vi "数字量输入配置.vi"() -> ()   [LabVIEW 2010] (continued)
                n7301 = property on="light_4" class="Bool (严格)"("Colors [4]"=w809) -> ()  [unwired: 2 in, 2 out]
                n7302 = property on="light_5" class="Bool (严格)"("Colors [4]"=w809) -> ()  [unwired: 2 in, 2 out]
                n7303 = property on="light_6" class="Bool (严格)"("Colors [4]"=w809) -> ()  [unwired: 2 in, 2 out]
                n7304 = property on="light_7" class="Bool (严格)"("Colors [4]"=w809) -> ()  [unwired: 2 in, 2 out]
                n7305 = property on="light_8" class="Bool (严格)"("Colors [4]"=w809) -> ()  [unwired: 2 in, 2 out]
                n7306 = property on="light_9" class="Bool (严格)"("Colors [4]"=w809) -> ()  [unwired: 2 in, 2 out]
                n7307 = property on="light_10" class="Bool (严格)"("Colors [4]"=w809) -> ()  [unwired: 2 in, 2 out]
                n7308 = property on="light_11" class="Bool (严格)"("Colors [4]"=w809) -> ()  [unwired: 2 in, 2 out]
                n7309 = property on="light_12" class="Bool (严格)"("Colors [4]"=w809) -> ()  [unwired: 2 in, 2 out]
                n7310 = property on="light_13" class="Bool (严格)"("Colors [4]"=w809) -> ()  [unwired: 2 in, 2 out]
                n7311 = property on="light_14" class="Bool (严格)"("Colors [4]"=w809) -> ()  [unwired: 2 in, 2 out]
                n7312 = property on="light_15" class="Bool (严格)"("Colors [4]"=w809) -> ()  [unwired: 2 in, 2 out]
                n7313 = property on="light_16" class="Bool (严格)"("Colors [4]"=w809) -> ()  [unwired: 2 in, 2 out]
                n7314 = property on="light_17" class="Bool (严格)"("Colors [4]"=w809) -> ()  [unwired: 2 in, 2 out]
                n7315 = property on="light_18" class="Bool (严格)"("Colors [4]"=w809) -> ()  [unwired: 2 in, 2 out]
                n7316 = property on="light_19" class="Bool (严格)"("Colors [4]"=w809) -> ()  [unwired: 2 in, 2 out]
                n7317 = property on="light_20" class="Bool (严格)"("Colors [4]"=w809) -> ()  [unwired: 2 in, 2 out]
                n7318 = property on="light_21" class="Bool (严格)"("Colors [4]"=w809) -> ()  [unwired: 2 in, 2 out]
                n7319 = property on="light_22" class="Bool (严格)"("Colors [4]"=w809) -> ()  [unwired: 2 in, 2 out]
                n7320 = property on="light_23" class="Bool (严格)"("Colors [4]"=w809) -> ()  [unwired: 2 in, 2 out]
                n7321 = property on="light_24" class="Bool (严格)"("Colors [4]"=w809) -> ()  [unwired: 2 in, 2 out]
                n7322 = property on="light_25" class="Bool (严格)"("Colors [4]"=w809) -> ()  [unwired: 2 in, 2 out]
                n7323 = property on="light_26" class="Bool (严格)"("Colors [4]"=w809) -> ()  [unwired: 2 in, 2 out]
                n7324 = property on="light_27" class="Bool (严格)"("Colors [4]"=w809) -> ()  [unwired: 2 in, 2 out]
                n7325 = property on="light_28" class="Bool (严格)"("Colors [4]"=w809) -> ()  [unwired: 2 in, 2 out]
                n7326 = property on="light_29" class="Bool (严格)"("Colors [4]"=w809) -> ()  [unwired: 2 in, 2 out]
                n7327 = property on="light_30" class="Bool (严格)"("Colors [4]"=w809) -> ()  [unwired: 2 in, 2 out]
                n7328 = property on="light_31" class="Bool (严格)"("Colors [4]"=w809) -> ()  [unwired: 2 in, 2 out]
                n7329 = property on="light_32" class="Bool (严格)"("Colors [4]"=w809) -> ()  [unwired: 2 in, 2 out]
                n7330 = property on="light_33" class="Bool (严格)"("Colors [4]"=w809) -> ()  [unwired: 2 in, 2 out]
                n7331 = property on="light_34" class="Bool (严格)"("Colors [4]"=w809) -> ()  [unwired: 2 in, 2 out]
                n7332 = property on="light_35" class="Bool (严格)"("Colors [4]"=w809) -> ()  [unwired: 2 in, 2 out]
                n7333 = property on="light_36" class="Bool (严格)"("Colors [4]"=w809) -> ()  [unwired: 2 in, 2 out]
                n7334 = property on="light_37" class="Bool (严格)"("Colors [4]"=w809) -> ()  [unwired: 2 in, 2 out]
                n7335 = property on="light_38" class="Bool (严格)"("Colors [4]"=w809) -> ()  [unwired: 2 in, 2 out]
                n7336 = property on="light_39" class="Bool (严格)"("Colors [4]"=w809) -> ()  [unwired: 2 in, 2 out]
                n7337 = property on="light_40" class="Bool (严格)"("Colors [4]"=w809) -> ()  [unwired: 2 in, 2 out]
                n7338 = property on="light_41" class="Bool (严格)"("Colors [4]"=w809) -> ()  [unwired: 2 in, 2 out]
                n7339 = property on="light_42" class="Bool (严格)"("Colors [4]"=w809) -> ()  [unwired: 2 in, 2 out]
                n7340 = property on="light_43" class="Bool (严格)"("Colors [4]"=w809) -> ()  [unwired: 2 in, 2 out]
                n7341 = property on="light_44" class="Bool (严格)"("Colors [4]"=w809) -> ()  [unwired: 2 in, 2 out]
                n7342 = property on="light_45" class="Bool (严格)"("Colors [4]"=w809) -> ()  [unwired: 2 in, 2 out]
                n7343 = property on="light_46" class="Bool (严格)"("Colors [4]"=w809) -> ()  [unwired: 2 in, 2 out]
                n7344 = property on="light_47" class="Bool (严格)"("Colors [4]"=w809) -> ()  [unwired: 2 in, 2 out]
                n7345 = property on="light_48" class="Bool (严格)"("Colors [4]"=w809) -> ()  [unwired: 2 in, 2 out]
                n7346 = property on="light_49" class="Bool (严格)"("Colors [4]"=w809) -> ()  [unwired: 2 in, 2 out]
                n7347 = property on="light_50" class="Bool (严格)"("Colors [4]"=w809) -> ()  [unwired: 2 in, 2 out]
                n7348 = property on="light_51" class="Bool (严格)"("Colors [4]"=w809) -> ()  [unwired: 2 in, 2 out]
                n7349 = property on="light_52" class="Bool (严格)"("Colors [4]"=w809) -> ()  [unwired: 2 in, 2 out]
                n7350 = property on="light_53" class="Bool (严格)"("Colors [4]"=w809) -> ()  [unwired: 2 in, 2 out]
                n7351 = property on="light_54" class="Bool (严格)"("Colors [4]"=w809) -> ()  [unwired: 2 in, 2 out]
                n7352 = property on="light_55" class="Bool (严格)"("Colors [4]"=w809) -> ()  [unwired: 2 in, 2 out]
                n7353 = property on="light_56" class="Bool (严格)"("Colors [4]"=w809) -> ()  [unwired: 2 in, 2 out]
                n7354 = property on="light_57" class="Bool (严格)"("Colors [4]"=w809) -> ()  [unwired: 2 in, 2 out]
                n7355 = property on="light_58" class="Bool (严格)"("Colors [4]"=w809) -> ()  [unwired: 2 in, 2 out]
                n7356 = property on="light_59" class="Bool (严格)"("Colors [4]"=w809) -> ()  [unwired: 2 in, 2 out]
                n7357 = property on="light_60" class="Bool (严格)"("Colors [4]"=w809) -> ()  [unwired: 2 in, 2 out]
                n7358 = property on="light_61" class="Bool (严格)"("Colors [4]"=w809) -> ()  [unwired: 2 in, 2 out]
                n7359 = property on="light_62" class="Bool (严格)"("Colors [4]"=w809) -> ()  [unwired: 2 in, 2 out]
                n7360 = property on="light_63" class="Bool (严格)"("Colors [4]"=w809) -> ()  [unwired: 2 in, 2 out]
                n7361 = property on="light_64" class="Bool (严格)"("Colors [4]"=w809) -> ()  [unwired: 2 in, 2 out]
                n7362 = property on="light_65" class="Bool (严格)"("Colors [4]"=w809) -> ()  [unwired: 2 in, 2 out]
                n7363 = property on="light_66" class="Bool (严格)"("Colors [4]"=w809) -> ()  [unwired: 2 in, 2 out]
                n7364 = property on="light_67" class="Bool (严格)"("Colors [4]"=w809) -> ()  [unwired: 2 in, 2 out]
                n7365 = property on="light_68" class="Bool (严格)"("Colors [4]"=w809) -> ()  [unwired: 2 in, 2 out]
                n7366 = property on="light_69" class="Bool (严格)"("Colors [4]"=w809) -> ()  [unwired: 2 in, 2 out]
                n7367 = property on="light_70" class="Bool (严格)"("Colors [4]"=w809) -> ()  [unwired: 2 in, 2 out]
                n7368 = property on="light_71" class="Bool (严格)"("Colors [4]"=w809) -> ()  [unwired: 2 in, 2 out]
                n7369 = property on="light_72" class="Bool (严格)"("Colors [4]"=w809) -> ()  [unwired: 2 in, 2 out]
                n7370 = property on="light_73" class="Bool (严格)"("Colors [4]"=w809) -> ()  [unwired: 2 in, 2 out]
                n7371 = property on="light_74" class="Bool (严格)"("Colors [4]"=w809) -> ()  [unwired: 2 in, 2 out]
                n7372 = property on="light_75" class="Bool (严格)"("Colors [4]"=w809) -> ()  [unwired: 2 in, 2 out]
                n7373 = property on="light_76" class="Bool (严格)"("Colors [4]"=w809) -> ()  [unwired: 2 in, 2 out]
                n7374 = property on="light_77" class="Bool (严格)"("Colors [4]"=w809) -> ()  [unwired: 2 in, 2 out]
                n7375 = property on="light_78" class="Bool (严格)"("Colors [4]"=w809) -> ()  [unwired: 2 in, 2 out]
                n7376 = property on="light_79" class="Bool (严格)"("Colors [4]"=w809) -> ()  [unwired: 2 in, 2 out]
                n7377 = property on="light_80" class="Bool (严格)"("Colors [4]"=w809) -> ()  [unwired: 2 in, 2 out]
                n7378 = Initialize Array("", 16 ("维数大小"), 4 ("维数大小")) -> (w808:string[][])
                n7379 = local write "D_IN_1"(w808) -> ()
                n7380 = local write "D_IN_2"(w808) -> ()
                n7381 = local write "D_IN_3"(w808) -> ()
                n7382 = local write "D_IN_4"(w808) -> ()
                n7383 = local write "D_IN_5"(w808) -> ()
              }
              frame #2 {
                n7384 = local read "保持输入"() -> (w810:bool)
                n7385 = case shown="假" w810 {
                  frame False {
                    n7386 = property on="保持输入" class="Bool (严格)"("DisabledEnum"=T1."Disabled and Grayed Out" ("禁用")) -> ()  [unwired: 2 in, 2 out]
                  }
                  frame True {
                    n7387 = local read "数组_选择?"() -> (w812:bool[][])
                    n7388 = for {
                      tunnel: w812 -> [w816] mode=indexing
                      i -> [w814]
                      stop <- w813 stop-if-true
                      n7389 = Or Array Elements(Boolean array=w816) -> (logical OR=w815:bool)
                      n7390 = case shown="真" w815 {
                        tunnel: w814 -> [_ w818]
                        tunnel: [FALSE w821] -> w813
                        frame False {
                        }
                        frame True {
                          n7391 = local write "同步_A1"(w818) -> ()
                          n7392 = Increment(x=w818) -> (x+1=w823:i32)
                          n7393 = Format Into String(format string="保持第%d组数据输入" ("格式字符串"), w823) -> (resulting string=w824:string)  [unwired: 2 in, 1 out]
                          n7394 = call "显示对话框信息2"("Message"=w824) -> ("是"=w819:bool)  [unwired: 9 in, 1 out]
                          n7395 = case shown="真" w819 {
                            tunnel: [FALSE w829] -> w821
                            tunnel: [T1."Enabled" ("禁用") w828] -> w820
                            tunnel: w818 -> [_ w827]
                            frame False {
                            }
                            frame True {
                              n7396 = stacked-sequence {
                                tunnel: [_ TRUE] -> w829
                                tunnel: [_ T1."Disabled and Grayed Out" ("禁用")] -> w828
                                tunnel: w827 -> [w830 _]
                                frame #0 {
                                n7397 = for {
                                N: 5 -> [_]
                                tunnel: w830 -> [w833]
                                i -> [w832]
                                n7398 = Not Equal?(x=w833, y=w832) -> (x != y?=w834:bool)
                                n7399 = case shown="真" w834 {
                                tunnel: w832 -> [_ w835]
                                frame False {
                                }
                                frame True {
                                n7400 = local read "数组_选择?"() -> (w839:bool[][])
                                n7401 = Initialize Array(FALSE, 16 ("维数大小")) -> (w836:bool[])
                                n7402 = Replace Array Subset(array=w839, new element=w836, index (row)=w835) -> (w840:bool[][])  [unwired: 1 in]
                                n7403 = local write "数组_选择?"(w840) -> ()
                                }
                                }
                                }
                                }
                                frame #1 {
                                }
                              }
                            }
                          }
                          n7404 = local write "保持输入"(w819) -> ()
                          n7405 = property on="btn_开始试验" class="Bool"("DisabledEnum"=w820) -> ()  [unwired: 2 in, 2 out]
                        }
                      }
                    }
                  }
                }
              }
              frame #3 {
                n7406 = local read "数组_选择?"() -> (w846:bool[][])
                n7407 = Or Array Elements(Boolean array=w846) -> (logical OR=w845:bool)
                n7408 = case shown="真" w845 {
                  tunnel: w844 -> [_ w849]
                  tunnel: w843 -> [_ w848]
                  frame False {
                    n7409 = call "显示对话框信息"("Message"="请选择数字量输入路数") -> ()  [unwired: 9 in, 2 out]
                  }
                  frame True {
                    n7410 = Send Notification(notification="DInput" ("通知"), notifier=w849, error in (no error)=w848) -> ()  [unwired: 2 out]
                  }
                }
              }
            }
          }
          event "保持输入": Value Change {
            n7411 = event-data() -> ()  [unwired: 1 in, 5 out]
            n7412 = property on="btn_开始试验" class="Bool"("DisabledEnum"=T1."Enabled" ("禁用")) -> ()  [unwired: 2 in, 2 out]
          }
          event "btn_全选": Value Change {
            w852 = TRUE ("单选_第41路")
            n7413 = event-data() -> ()  [unwired: 1 in, 5 out]
            n7414 = local write "单选_第1路"(w852) -> ()
            n7415 = local write "单选_第2路"(w852) -> ()
            n7416 = local write "单选_第3路"(w852) -> ()
            n7417 = local write "单选_第4路"(w852) -> ()
            n7418 = local write "单选_第5路"(w852) -> ()
            n7419 = local write "单选_第6路"(w852) -> ()
            n7420 = local write "单选_第7路"(w852) -> ()
            n7421 = local write "单选_第8路"(w852) -> ()
            n7422 = local write "单选_第9路"(w852) -> ()
            n7423 = local write "单选_第10路"(w852) -> ()
            n7424 = local write "单选_第11路"(w852) -> ()
            n7425 = local write "单选_第12路"(w852) -> ()
            n7426 = local write "单选_第13路"(w852) -> ()
            n7427 = local write "单选_第14路"(w852) -> ()
            n7428 = local write "单选_第15路"(w852) -> ()
            n7429 = local write "单选_第16路"(w852) -> ()
            n7430 = local write "单选_第17路"(w852) -> ()
            n7431 = local write "单选_第18路"(w852) -> ()
            n7432 = local write "单选_第19路"(w852) -> ()
            n7433 = local write "单选_第20路"(w852) -> ()
            n7434 = local write "单选_第21路"(w852) -> ()
            n7435 = local write "单选_第22路"(w852) -> ()
            n7436 = local write "单选_第23路"(w852) -> ()
            n7437 = local write "单选_第24路"(w852) -> ()
            n7438 = local write "单选_第25路"(w852) -> ()
            n7439 = local write "单选_第26路"(w852) -> ()
            n7440 = local write "单选_第27路"(w852) -> ()
            n7441 = local write "单选_第28路"(w852) -> ()
            n7442 = local write "单选_第29路"(w852) -> ()
            n7443 = local write "单选_第30路"(w852) -> ()
            n7444 = local write "单选_第31路"(w852) -> ()
            n7445 = local write "单选_第32路"(w852) -> ()
            n7446 = local write "单选_第33路"(w852) -> ()
            n7447 = local write "单选_第34路"(w852) -> ()
            n7448 = local write "单选_第35路"(w852) -> ()
            n7449 = local write "单选_第36路"(w852) -> ()
            n7450 = local write "单选_第37路"(w852) -> ()
            n7451 = local write "单选_第38路"(w852) -> ()
            n7452 = local write "单选_第39路"(w852) -> ()
            n7453 = local write "单选_第40路"(w852) -> ()
            n7454 = local write "单选_第41路"(w852) -> ()
            n7455 = local write "单选_第42路"(w852) -> ()
            n7456 = local write "单选_第43路"(w852) -> ()
            n7457 = local write "单选_第44路"(w852) -> ()
            n7458 = local write "单选_第45路"(w852) -> ()
            n7459 = local write "单选_第46路"(w852) -> ()
            n7460 = local write "单选_第47路"(w852) -> ()
            n7461 = local write "单选_第48路"(w852) -> ()
            n7462 = local write "单选_第49路"(w852) -> ()
            n7463 = local write "单选_第50路"(w852) -> ()
            n7464 = local write "单选_第51路"(w852) -> ()
            n7465 = local write "单选_第52路"(w852) -> ()
            n7466 = local write "单选_第53路"(w852) -> ()
            n7467 = local write "单选_第54路"(w852) -> ()
            n7468 = local write "单选_第55路"(w852) -> ()
            n7469 = local write "单选_第56路"(w852) -> ()
            n7470 = local write "单选_第57路"(w852) -> ()
            n7471 = local write "单选_第58路"(w852) -> ()
            n7472 = local write "单选_第59路"(w852) -> ()
            n7473 = local write "单选_第60路"(w852) -> ()
            n7474 = local write "单选_第61路"(w852) -> ()
            n7475 = local write "单选_第62路"(w852) -> ()
            n7476 = local write "单选_第63路"(w852) -> ()
            n7477 = local write "单选_第64路"(w852) -> ()
            n7478 = local write "单选_第71路"(w852) -> ()
            n7479 = local write "单选_第79路"(w852) -> ()
            n7480 = local write "单选_第65路"(w852) -> ()
            n7481 = local write "单选_第66路"(w852) -> ()
            n7482 = local write "单选_第67路"(w852) -> ()
            n7483 = local write "单选_第68路"(w852) -> ()
            n7484 = local write "单选_第69路"(w852) -> ()
            n7485 = local write "单选_第70路"(w852) -> ()
            n7486 = local write "单选_第72路"(w852) -> ()
            n7487 = local write "单选_第73路"(w852) -> ()
            n7488 = local write "单选_第74路"(w852) -> ()
            n7489 = local write "单选_第75路"(w852) -> ()
            n7490 = local write "单选_第76路"(w852) -> ()
            n7491 = local write "单选_第77路"(w852) -> ()
            n7492 = local write "单选_第78路"(w852) -> ()
            n7493 = local write "单选_第80路"(w852) -> ()
          }
          event "btn_反选": Value Change {
            n7494 = event-data() -> ()  [unwired: 1 in, 5 out]
            n7495 = local read "单选_第1路"() -> (w1012:bool)
            n7496 = local read "单选_第2路"() -> (w1010:bool)
            n7497 = local read "单选_第3路"() -> (w1008:bool)
            n7498 = local read "单选_第4路"() -> (w1006:bool)
            n7499 = local read "单选_第5路"() -> (w1004:bool)
            n7500 = local read "单选_第6路"() -> (w1002:bool)
            n7501 = local read "单选_第7路"() -> (w1001:bool)
            n7502 = local read "单选_第8路"() -> (w1000:bool)
            n7503 = local read "单选_第9路"() -> (w999:bool)
            n7504 = local read "单选_第10路"() -> (w998:bool)
            n7505 = local read "单选_第11路"() -> (w997:bool)
            n7506 = local read "单选_第12路"() -> (w996:bool)
            n7507 = local read "单选_第13路"() -> (w995:bool)
            n7508 = local read "单选_第14路"() -> (w994:bool)
            n7509 = local read "单选_第15路"() -> (w993:bool)
            n7510 = local read "单选_第16路"() -> (w992:bool)
            n7511 = local read "单选_第17路"() -> (w991:bool)
            n7512 = local read "单选_第18路"() -> (w990:bool)
            n7513 = local read "单选_第19路"() -> (w989:bool)
            n7514 = local read "单选_第20路"() -> (w988:bool)
            n7515 = local read "单选_第21路"() -> (w987:bool)
            n7516 = local read "单选_第22路"() -> (w986:bool)
            n7517 = local read "单选_第23路"() -> (w985:bool)
            n7518 = local read "单选_第24路"() -> (w984:bool)
            n7519 = local read "单选_第25路"() -> (w983:bool)
            n7520 = local read "单选_第26路"() -> (w982:bool)
            n7521 = local read "单选_第27路"() -> (w981:bool)
            n7522 = local read "单选_第28路"() -> (w980:bool)
            n7523 = local read "单选_第29路"() -> (w979:bool)
            n7524 = local read "单选_第30路"() -> (w978:bool)
            n7525 = local read "单选_第31路"() -> (w977:bool)
            n7526 = local read "单选_第32路"() -> (w976:bool)
            n7527 = local read "单选_第33路"() -> (w975:bool)
            n7528 = local read "单选_第34路"() -> (w974:bool)
            n7529 = local read "单选_第35路"() -> (w973:bool)
            n7530 = local read "单选_第36路"() -> (w972:bool)
            n7531 = local read "单选_第37路"() -> (w971:bool)
            n7532 = local read "单选_第38路"() -> (w970:bool)
            n7533 = local read "单选_第39路"() -> (w969:bool)
            n7534 = local read "单选_第40路"() -> (w968:bool)
            n7535 = Not(x=w1012) -> (.not. x?=w1011:bool)
            n7536 = Not(x=w1010) -> (.not. x?=w1009:bool)
            n7537 = Not(x=w1008) -> (.not. x?=w1007:bool)
            n7538 = Not(x=w1006) -> (.not. x?=w1005:bool)
            n7539 = Not(x=w1004) -> (.not. x?=w1003:bool)
            n7540 = Not(x=w1002) -> (.not. x?=w967:bool)
            n7541 = Not(x=w1001) -> (.not. x?=w966:bool)
            n7542 = Not(x=w1000) -> (.not. x?=w965:bool)
            n7543 = Not(x=w999) -> (.not. x?=w964:bool)
            n7544 = Not(x=w998) -> (.not. x?=w963:bool)
            n7545 = Not(x=w997) -> (.not. x?=w962:bool)
            n7546 = Not(x=w996) -> (.not. x?=w961:bool)
            n7547 = Not(x=w995) -> (.not. x?=w960:bool)
            n7548 = Not(x=w994) -> (.not. x?=w959:bool)
            n7549 = Not(x=w993) -> (.not. x?=w958:bool)
            n7550 = Not(x=w992) -> (.not. x?=w957:bool)
            n7551 = Not(x=w991) -> (.not. x?=w956:bool)
            n7552 = Not(x=w990) -> (.not. x?=w955:bool)
            n7553 = Not(x=w989) -> (.not. x?=w954:bool)
            n7554 = Not(x=w988) -> (.not. x?=w953:bool)
            n7555 = Not(x=w987) -> (.not. x?=w952:bool)
            n7556 = Not(x=w986) -> (.not. x?=w951:bool)
            n7557 = Not(x=w985) -> (.not. x?=w950:bool)
            n7558 = Not(x=w984) -> (.not. x?=w949:bool)
            n7559 = Not(x=w983) -> (.not. x?=w948:bool)
            n7560 = Not(x=w982) -> (.not. x?=w947:bool)
            n7561 = Not(x=w981) -> (.not. x?=w946:bool)
            n7562 = Not(x=w980) -> (.not. x?=w945:bool)
            n7563 = Not(x=w979) -> (.not. x?=w944:bool)
            n7564 = Not(x=w978) -> (.not. x?=w943:bool)
            n7565 = Not(x=w977) -> (.not. x?=w942:bool)
            n7566 = Not(x=w976) -> (.not. x?=w941:bool)
            n7567 = Not(x=w975) -> (.not. x?=w940:bool)
            n7568 = Not(x=w974) -> (.not. x?=w939:bool)
            n7569 = Not(x=w973) -> (.not. x?=w938:bool)
            n7570 = Not(x=w972) -> (.not. x?=w937:bool)
            n7571 = Not(x=w971) -> (.not. x?=w936:bool)
            n7572 = Not(x=w970) -> (.not. x?=w935:bool)
            n7573 = Not(x=w969) -> (.not. x?=w934:bool)
            n7574 = Not(x=w968) -> (.not. x?=w933:bool)
            n7575 = local write "单选_第1路"(w1011) -> ()
            n7576 = local write "单选_第2路"(w1009) -> ()
            n7577 = local write "单选_第3路"(w1007) -> ()
            n7578 = local write "单选_第4路"(w1005) -> ()
            n7579 = local write "单选_第5路"(w1003) -> ()
            n7580 = local write "单选_第6路"(w967) -> ()
            n7581 = local write "单选_第7路"(w966) -> ()
            n7582 = local write "单选_第8路"(w965) -> ()
            n7583 = local write "单选_第9路"(w964) -> ()
            n7584 = local write "单选_第10路"(w963) -> ()
            n7585 = local write "单选_第11路"(w962) -> ()
            n7586 = local write "单选_第12路"(w961) -> ()
            n7587 = local write "单选_第13路"(w960) -> ()
            n7588 = local write "单选_第14路"(w959) -> ()
            n7589 = local write "单选_第15路"(w958) -> ()
            n7590 = local write "单选_第16路"(w957) -> ()
            n7591 = local write "单选_第17路"(w956) -> ()
            n7592 = local write "单选_第18路"(w955) -> ()
            n7593 = local write "单选_第19路"(w954) -> ()
            n7594 = local write "单选_第20路"(w953) -> ()
            n7595 = local write "单选_第21路"(w952) -> ()
            n7596 = local write "单选_第22路"(w951) -> ()
            n7597 = local write "单选_第23路"(w950) -> ()
            n7598 = local write "单选_第24路"(w949) -> ()
            n7599 = local write "单选_第25路"(w948) -> ()
            n7600 = local write "单选_第26路"(w947) -> ()
            n7601 = local write "单选_第27路"(w946) -> ()
            n7602 = local write "单选_第28路"(w945) -> ()
            n7603 = local write "单选_第29路"(w944) -> ()
            n7604 = local write "单选_第30路"(w943) -> ()
            n7605 = local write "单选_第31路"(w942) -> ()
            n7606 = local write "单选_第32路"(w941) -> ()
            n7607 = local write "单选_第33路"(w940) -> ()
            n7608 = local write "单选_第34路"(w939) -> ()
            n7609 = local write "单选_第35路"(w938) -> ()
            n7610 = local write "单选_第36路"(w937) -> ()
            n7611 = local write "单选_第37路"(w936) -> ()
            n7612 = local write "单选_第38路"(w935) -> ()
            n7613 = local write "单选_第39路"(w934) -> ()
            n7614 = local write "单选_第40路"(w933) -> ()
            n7615 = local read "单选_第71路"() -> (w902:bool)
            n7616 = local read "单选_第79路"() -> (w894:bool)
            n7617 = local read "单选_第41路"() -> (w932:bool)
            n7618 = local read "单选_第42路"() -> (w931:bool)
            n7619 = local read "单选_第43路"() -> (w930:bool)
            n7620 = local read "单选_第44路"() -> (w929:bool)
            n7621 = local read "单选_第45路"() -> (w928:bool)
            n7622 = local read "单选_第46路"() -> (w927:bool)
            n7623 = local read "单选_第47路"() -> (w926:bool)
            n7624 = local read "单选_第48路"() -> (w925:bool)
            n7625 = local read "单选_第49路"() -> (w924:bool)
            n7626 = local read "单选_第50路"() -> (w923:bool)
            n7627 = local read "单选_第51路"() -> (w922:bool)
            n7628 = local read "单选_第52路"() -> (w921:bool)
            n7629 = local read "单选_第53路"() -> (w920:bool)
            n7630 = local read "单选_第54路"() -> (w919:bool)
            n7631 = local read "单选_第55路"() -> (w918:bool)
            n7632 = local read "单选_第56路"() -> (w917:bool)
            n7633 = local read "单选_第57路"() -> (w916:bool)
            n7634 = local read "单选_第58路"() -> (w915:bool)
            n7635 = local read "单选_第59路"() -> (w914:bool)
            n7636 = local read "单选_第60路"() -> (w913:bool)
            n7637 = local read "单选_第61路"() -> (w912:bool)
            n7638 = local read "单选_第62路"() -> (w911:bool)
            n7639 = local read "单选_第63路"() -> (w910:bool)
            n7640 = local read "单选_第64路"() -> (w909:bool)
            n7641 = local read "单选_第65路"() -> (w908:bool)
            n7642 = local read "单选_第66路"() -> (w907:bool)
            n7643 = local read "单选_第67路"() -> (w906:bool)
            n7644 = local read "单选_第68路"() -> (w905:bool)
            n7645 = local read "单选_第69路"() -> (w904:bool)
            n7646 = local read "单选_第70路"() -> (w903:bool)
            n7647 = local read "单选_第72路"() -> (w901:bool)
            n7648 = local read "单选_第73路"() -> (w900:bool)
            n7649 = local read "单选_第74路"() -> (w899:bool)
            n7650 = local read "单选_第75路"() -> (w898:bool)
            n7651 = local read "单选_第76路"() -> (w897:bool)
            n7652 = local read "单选_第77路"() -> (w896:bool)
            n7653 = local read "单选_第78路"() -> (w895:bool)
            n7654 = local read "单选_第80路"() -> (w893:bool)
            n7655 = Not(x=w932) -> (.not. x?=w892:bool)
            n7656 = Not(x=w931) -> (.not. x?=w891:bool)
            n7657 = Not(x=w930) -> (.not. x?=w890:bool)
            n7658 = Not(x=w929) -> (.not. x?=w889:bool)
            n7659 = Not(x=w928) -> (.not. x?=w888:bool)
            n7660 = Not(x=w927) -> (.not. x?=w887:bool)
            n7661 = Not(x=w926) -> (.not. x?=w886:bool)
            n7662 = Not(x=w925) -> (.not. x?=w885:bool)
            n7663 = Not(x=w924) -> (.not. x?=w884:bool)
            n7664 = Not(x=w923) -> (.not. x?=w883:bool)
            n7665 = Not(x=w922) -> (.not. x?=w882:bool)
            n7666 = Not(x=w921) -> (.not. x?=w881:bool)
            n7667 = Not(x=w920) -> (.not. x?=w880:bool)
            n7668 = Not(x=w919) -> (.not. x?=w879:bool)
            n7669 = Not(x=w918) -> (.not. x?=w878:bool)
            n7670 = Not(x=w917) -> (.not. x?=w877:bool)
            n7671 = Not(x=w916) -> (.not. x?=w876:bool)
            n7672 = Not(x=w915) -> (.not. x?=w875:bool)
            n7673 = Not(x=w914) -> (.not. x?=w874:bool)
            n7674 = Not(x=w913) -> (.not. x?=w873:bool)
            n7675 = Not(x=w912) -> (.not. x?=w872:bool)
            n7676 = Not(x=w911) -> (.not. x?=w871:bool)
            n7677 = Not(x=w910) -> (.not. x?=w870:bool)
            n7678 = Not(x=w909) -> (.not. x?=w869:bool)
            n7679 = Not(x=w908) -> (.not. x?=w868:bool)
            n7680 = Not(x=w907) -> (.not. x?=w867:bool)
            n7681 = Not(x=w906) -> (.not. x?=w866:bool)
            n7682 = Not(x=w905) -> (.not. x?=w865:bool)
            n7683 = Not(x=w904) -> (.not. x?=w864:bool)
            n7684 = Not(x=w903) -> (.not. x?=w863:bool)
            n7685 = Not(x=w902) -> (.not. x?=w862:bool)
            n7686 = Not(x=w901) -> (.not. x?=w861:bool)
            n7687 = Not(x=w900) -> (.not. x?=w860:bool)
            n7688 = Not(x=w899) -> (.not. x?=w859:bool)
            n7689 = Not(x=w898) -> (.not. x?=w858:bool)
            n7690 = Not(x=w897) -> (.not. x?=w857:bool)
            n7691 = Not(x=w896) -> (.not. x?=w856:bool)
            n7692 = Not(x=w895) -> (.not. x?=w855:bool)
            n7693 = Not(x=w894) -> (.not. x?=w854:bool)
            n7694 = Not(x=w893) -> (.not. x?=w853:bool)
            n7695 = local write "单选_第71路"(w862) -> ()
            n7696 = local write "单选_第79路"(w854) -> ()
            n7697 = local write "单选_第41路"(w892) -> ()
            n7698 = local write "单选_第42路"(w891) -> ()
            n7699 = local write "单选_第43路"(w890) -> ()
            n7700 = local write "单选_第44路"(w889) -> ()
            n7701 = local write "单选_第45路"(w888) -> ()
            n7702 = local write "单选_第46路"(w887) -> ()
            n7703 = local write "单选_第47路"(w886) -> ()
            n7704 = local write "单选_第48路"(w885) -> ()
            n7705 = local write "单选_第49路"(w884) -> ()
            n7706 = local write "单选_第50路"(w883) -> ()
            n7707 = local write "单选_第51路"(w882) -> ()
            n7708 = local write "单选_第52路"(w881) -> ()
            n7709 = local write "单选_第53路"(w880) -> ()
            n7710 = local write "单选_第54路"(w879) -> ()
            n7711 = local write "单选_第55路"(w878) -> ()
            n7712 = local write "单选_第56路"(w877) -> ()
            n7713 = local write "单选_第57路"(w876) -> ()
            n7714 = local write "单选_第58路"(w875) -> ()
            n7715 = local write "单选_第59路"(w874) -> ()
            n7716 = local write "单选_第60路"(w873) -> ()
            n7717 = local write "单选_第61路"(w872) -> ()
            n7718 = local write "单选_第62路"(w871) -> ()
            n7719 = local write "单选_第63路"(w870) -> ()
            n7720 = local write "单选_第64路"(w869) -> ()
            n7721 = local write "单选_第65路"(w868) -> ()
            n7722 = local write "单选_第66路"(w867) -> ()
            n7723 = local write "单选_第67路"(w866) -> ()
            n7724 = local write "单选_第68路"(w865) -> ()
            n7725 = local write "单选_第69路"(w864) -> ()
            n7726 = local write "单选_第70路"(w863) -> ()
            n7727 = local write "单选_第72路"(w861) -> ()
            n7728 = local write "单选_第73路"(w860) -> ()
            n7729 = local write "单选_第74路"(w859) -> ()
            n7730 = local write "单选_第75路"(w858) -> ()
            n7731 = local write "单选_第76路"(w857) -> ()
            n7732 = local write "单选_第77路"(w856) -> ()
            n7733 = local write "单选_第78路"(w855) -> ()
            n7734 = local write "单选_第80路"(w853) -> ()
          }
          event "btn_置1": Value Change {
            w1013 = enum16{"0", "1"}."1" ("输入值_41")
            n7735 = event-data() -> ()  [unwired: 1 in, 5 out]
            n7736 = local write "输入值_1"(w1013) -> ()
            n7737 = local write "输入值_2"(w1013) -> ()
            n7738 = local write "输入值_3"(w1013) -> ()
            n7739 = local write "输入值_4"(w1013) -> ()
            n7740 = local write "输入值_5"(w1013) -> ()
            n7741 = local write "输入值_6"(w1013) -> ()
            n7742 = local write "输入值_7"(w1013) -> ()
            n7743 = local write "输入值_8"(w1013) -> ()
            n7744 = local write "输入值_9"(w1013) -> ()
            n7745 = local write "输入值_10"(w1013) -> ()
            n7746 = local write "输入值_11"(w1013) -> ()
            n7747 = local write "输入值_12"(w1013) -> ()
            n7748 = local write "输入值_13"(w1013) -> ()
            n7749 = local write "输入值_14"(w1013) -> ()
            n7750 = local write "输入值_15"(w1013) -> ()
            n7751 = local write "输入值_16"(w1013) -> ()
            n7752 = local write "输入值_17"(w1013) -> ()
            n7753 = local write "输入值_18"(w1013) -> ()
            n7754 = local write "输入值_19"(w1013) -> ()
            n7755 = local write "输入值_20"(w1013) -> ()
            n7756 = local write "输入值_21"(w1013) -> ()
            n7757 = local write "输入值_22"(w1013) -> ()
            n7758 = local write "输入值_23"(w1013) -> ()
            n7759 = local write "输入值_24"(w1013) -> ()
            n7760 = local write "输入值_25"(w1013) -> ()
            n7761 = local write "输入值_26"(w1013) -> ()
            n7762 = local write "输入值_27"(w1013) -> ()
            n7763 = local write "输入值_28"(w1013) -> ()
            n7764 = local write "输入值_29"(w1013) -> ()
            n7765 = local write "输入值_30"(w1013) -> ()
            n7766 = local write "输入值_31"(w1013) -> ()
            n7767 = local write "输入值_32"(w1013) -> ()
            n7768 = local write "输入值_33"(w1013) -> ()
            n7769 = local write "输入值_34"(w1013) -> ()
            n7770 = local write "输入值_35"(w1013) -> ()
            n7771 = local write "输入值_36"(w1013) -> ()
            n7772 = local write "输入值_37"(w1013) -> ()
            n7773 = local write "输入值_38"(w1013) -> ()
            n7774 = local write "输入值_39"(w1013) -> ()
            n7775 = local write "输入值_40"(w1013) -> ()
            n7776 = local write "输入值_41"(w1013) -> ()
            n7777 = local write "输入值_42"(w1013) -> ()
            n7778 = local write "输入值_43"(w1013) -> ()
            n7779 = local write "输入值_44"(w1013) -> ()
            n7780 = local write "输入值_45"(w1013) -> ()
            n7781 = local write "输入值_46"(w1013) -> ()
            n7782 = local write "输入值_47"(w1013) -> ()
            n7783 = local write "输入值_48"(w1013) -> ()
            n7784 = local write "输入值_49"(w1013) -> ()
            n7785 = local write "输入值_50"(w1013) -> ()
            n7786 = local write "输入值_51"(w1013) -> ()
            n7787 = local write "输入值_52"(w1013) -> ()
            n7788 = local write "输入值_53"(w1013) -> ()
            n7789 = local write "输入值_54"(w1013) -> ()
            n7790 = local write "输入值_55"(w1013) -> ()
            n7791 = local write "输入值_56"(w1013) -> ()
            n7792 = local write "输入值_57"(w1013) -> ()
            n7793 = local write "输入值_58"(w1013) -> ()
            n7794 = local write "输入值_59"(w1013) -> ()
            n7795 = local write "输入值_60"(w1013) -> ()
            n7796 = local write "输入值_61"(w1013) -> ()
            n7797 = local write "输入值_62"(w1013) -> ()
            n7798 = local write "输入值_63"(w1013) -> ()
            n7799 = local write "输入值_64"(w1013) -> ()
            n7800 = local write "输入值_65"(w1013) -> ()
            n7801 = local write "输入值_66"(w1013) -> ()
            n7802 = local write "输入值_67"(w1013) -> ()
            n7803 = local write "输入值_68"(w1013) -> ()
            n7804 = local write "输入值_69"(w1013) -> ()
            n7805 = local write "输入值_70"(w1013) -> ()
            n7806 = local write "输入值_71"(w1013) -> ()
            n7807 = local write "输入值_72"(w1013) -> ()
            n7808 = local write "输入值_73"(w1013) -> ()
            n7809 = local write "输入值_74"(w1013) -> ()
            n7810 = local write "输入值_75"(w1013) -> ()
            n7811 = local write "输入值_76"(w1013) -> ()
            n7812 = local write "输入值_77"(w1013) -> ()
            n7813 = local write "输入值_78"(w1013) -> ()
            n7814 = local write "输入值_79"(w1013) -> ()
            n7815 = local write "输入值_80"(w1013) -> ()
          }
          event "btn_置0": Value Change {
            w1014 = enum16{"0", "1"}."0" ("输入值_41")
            n7816 = event-data() -> ()  [unwired: 1 in, 5 out]
            n7817 = local write "输入值_1"(w1014) -> ()
            n7818 = local write "输入值_2"(w1014) -> ()
            n7819 = local write "输入值_3"(w1014) -> ()
            n7820 = local write "输入值_4"(w1014) -> ()
            n7821 = local write "输入值_5"(w1014) -> ()
            n7822 = local write "输入值_6"(w1014) -> ()
            n7823 = local write "输入值_7"(w1014) -> ()
            n7824 = local write "输入值_8"(w1014) -> ()
            n7825 = local write "输入值_9"(w1014) -> ()
            n7826 = local write "输入值_10"(w1014) -> ()
            n7827 = local write "输入值_11"(w1014) -> ()
            n7828 = local write "输入值_12"(w1014) -> ()
            n7829 = local write "输入值_13"(w1014) -> ()
            n7830 = local write "输入值_14"(w1014) -> ()
            n7831 = local write "输入值_15"(w1014) -> ()
            n7832 = local write "输入值_16"(w1014) -> ()
            n7833 = local write "输入值_17"(w1014) -> ()
            n7834 = local write "输入值_18"(w1014) -> ()
            n7835 = local write "输入值_19"(w1014) -> ()
            n7836 = local write "输入值_20"(w1014) -> ()
            n7837 = local write "输入值_21"(w1014) -> ()
            n7838 = local write "输入值_22"(w1014) -> ()
            n7839 = local write "输入值_23"(w1014) -> ()
            n7840 = local write "输入值_24"(w1014) -> ()
            n7841 = local write "输入值_25"(w1014) -> ()
            n7842 = local write "输入值_26"(w1014) -> ()
            n7843 = local write "输入值_27"(w1014) -> ()
            n7844 = local write "输入值_28"(w1014) -> ()
            n7845 = local write "输入值_29"(w1014) -> ()
            n7846 = local write "输入值_30"(w1014) -> ()
            n7847 = local write "输入值_31"(w1014) -> ()
            n7848 = local write "输入值_32"(w1014) -> ()
            n7849 = local write "输入值_33"(w1014) -> ()
            n7850 = local write "输入值_34"(w1014) -> ()
            n7851 = local write "输入值_35"(w1014) -> ()
            n7852 = local write "输入值_36"(w1014) -> ()
            n7853 = local write "输入值_37"(w1014) -> ()
            n7854 = local write "输入值_38"(w1014) -> ()
            n7855 = local write "输入值_39"(w1014) -> ()
            n7856 = local write "输入值_40"(w1014) -> ()
            n7857 = local write "输入值_41"(w1014) -> ()
            n7858 = local write "输入值_42"(w1014) -> ()
            n7859 = local write "输入值_43"(w1014) -> ()
            n7860 = local write "输入值_44"(w1014) -> ()
            n7861 = local write "输入值_45"(w1014) -> ()
            n7862 = local write "输入值_46"(w1014) -> ()
            n7863 = local write "输入值_47"(w1014) -> ()
            n7864 = local write "输入值_48"(w1014) -> ()
            n7865 = local write "输入值_49"(w1014) -> ()
            n7866 = local write "输入值_50"(w1014) -> ()
            n7867 = local write "输入值_51"(w1014) -> ()
            n7868 = local write "输入值_52"(w1014) -> ()
            n7869 = local write "输入值_53"(w1014) -> ()
            n7870 = local write "输入值_54"(w1014) -> ()
            n7871 = local write "输入值_55"(w1014) -> ()
            n7872 = local write "输入值_56"(w1014) -> ()
            n7873 = local write "输入值_57"(w1014) -> ()
            n7874 = local write "输入值_58"(w1014) -> ()
            n7875 = local write "输入值_59"(w1014) -> ()
            n7876 = local write "输入值_60"(w1014) -> ()
            n7877 = local write "输入值_61"(w1014) -> ()
            n7878 = local write "输入值_62"(w1014) -> ()
            n7879 = local write "输入值_63"(w1014) -> ()
            n7880 = local write "输入值_64"(w1014) -> ()
            n7881 = local write "输入值_65"(w1014) -> ()
            n7882 = local write "输入值_66"(w1014) -> ()
            n7883 = local write "输入值_67"(w1014) -> ()
            n7884 = local write "输入值_68"(w1014) -> ()
            n7885 = local write "输入值_69"(w1014) -> ()
            n7886 = local write "输入值_70"(w1014) -> ()
            n7887 = local write "输入值_71"(w1014) -> ()
            n7888 = local write "输入值_72"(w1014) -> ()
            n7889 = local write "输入值_73"(w1014) -> ()
            n7890 = local write "输入值_74"(w1014) -> ()
            n7891 = local write "输入值_75"(w1014) -> ()
            n7892 = local write "输入值_76"(w1014) -> ()
            n7893 = local write "输入值_77"(w1014) -> ()
            n7894 = local write "输入值_78"(w1014) -> ()
            n7895 = local write "输入值_79"(w1014) -> ()
            n7896 = local write "输入值_80"(w1014) -> ()
          }
        }
      }
      n7897 = Obtain Notifier(name (unnamed)=w203, notification data type=w203) -> (notifier out=w207:refnum<notifier>, error out=w206:errorcluster)  [unwired: 2 in, 1 out]
      n7898 = Obtain Notifier(name (unnamed)=w194, notification data type=w194) -> (notifier out=w193:refnum<notifier>)  [unwired: 2 in, 2 out]
      n7899 = while {
        tunnel: w207 -> [w460]
        tunnel: w206 -> [w459]
        tunnel: [w458] -> w205
        tunnel: [w457] -> w204
        tunnel: w193 -> [w456]
        stop <- w462 stop-if-true
        n7900 = Wait Until Next ms Multiple(millisecond multiple=u32 5 ("毫秒倍数")) -> ()  [unwired: 1 out]
        n7901 = Wait on Notification(notifier=w460, timeout in ms (-1)=20 ("超时毫秒(-1)"), error in (no error)=w459) -> (notifier out=w458:refnum<notifier>, notification=w466:string, error out=w457:errorcluster)  [unwired: 1 in, 1 out]
        n7902 = Equal?(x=w466, y="DInput" ("通知")) -> (x = y?=w461:bool)
        n7903 = case shown="真" w461 {
          tunnel: w456 -> [_ w467]
          frame False {
          }
          frame True {
            n7904 = while {
              tunnel: w467 -> [w468]
              stop <- w469 stop-if-true
              n7905 = stacked-sequence {
                tunnel: [w471 _] -> w469
                tunnel: w468 -> [_ w482]
                frame #0 {
                  n7906 = local read "保持输入"() -> (w474:bool)
                  n7907 = case shown="假" w474 {
                    selector: w474 -> [_ w480]
                    tunnel: [w477 w479] -> w473
                    frame False {
                      n7908 = local read "同步_A1"() -> (w476:i32)
                      n7909 = Equal?(x=w476, y=5) -> (x = y?=w477:bool)
                    }
                    frame True {
                      n7910 = Not(x=w480) -> (.not. x?=w479:bool)
                    }
                  }
                  n7911 = local read "关闭？"() -> (w472:bool)
                  n7912 = Or(x=w473, y=w472) -> (x .or. y?=w471:bool)
                  n7913 = case shown="真" w471 {
                    frame False {
                    }
                    frame True {
                      n7914 = property on="保持输入" class="Bool (严格)"("DisabledEnum"=T1."Enabled" ("禁用")) -> ()  [unwired: 2 in, 2 out]
                    }
                  }
                }
                frame #1 {
                  n7915 = local read "保持输入"() -> (w483:bool)
                  n7916 = local read "同步_A1"() -> (w481:i32)
                  n7917 = case shown="假" w483 {
                    tunnel: w481 -> [w492 _]
                    tunnel: [w487 TRUE] -> w484
                    frame False {
                      n7918 = local read "同步_A2"() -> (w491:i32)
                      n7919 = Equal?(x=w492, y=w491) -> (x = y?=w489:bool)
                      n7920 = Less?(x=w491, y=5) -> (x < y?=w488:bool)
                      n7921 = And(x=w489, y=w488) -> (x .and. y?=w487:bool)
                    }
                    frame True {
                    }
                  }
                  n7922 = local read "数组_选择?"() -> (w486:bool[][])
                  n7923 = local read "数组_输入值"() -> (w485:enum16{"0", "1"}[][])
                  n7924 = case shown="真" w484 {
                    tunnel: w486 -> [_ w497]
                    tunnel: w481 -> [_ w494]
                    tunnel: w485 -> [_ w499]
                    tunnel: w482 -> [_ w495]
                    frame False {
                    }
                    frame True {
                      n7925 = Index Array(array=w497, index (row)=w494) -> (element=w496:bool[])  [unwired: 1 in]
                      n7926 = Index Array(array=w499, index (row)=w494) -> (element=w498:enum16{"0", "1"}[])  [unwired: 1 in]
                      n7927 = Or Array Elements(Boolean array=w496) -> (logical OR=w500:bool)
                      n7928 = case shown="真" w500 {
                        tunnel: w498 -> [_ w509]
                        tunnel: w494 -> [_ w510]
                        tunnel: w495 -> [_ w507]
                        frame False {
                          n7929 = local read "保持输入"() -> (w501:bool)
                          n7930 = case shown="假" w501 {
                            frame False {
                              n7931 = local read "同步_A1"() -> (w504:i32)
                              n7932 = local read "同步_A2"() -> (w502:i32)
                              n7933 = Increment(x=w502) -> (x+1=w503:i32)
                              n7934 = Increment(x=w504) -> (x+1=w505:i32)
                              n7935 = local write "同步_A2"(w503) -> ()
                              n7936 = local write "同步_A1"(w505) -> ()
                            }
                            frame True {
                            }
                          }
                        }
                        frame True {
                          n7937 = local read "CAN端口"() -> (w511:u16)
                          n7938 = Increment(x=w510) -> (x+1=w508:i32)
                          n7939 = call "16路数字量输入.vi"("第几组数据"=w508, "CAN端口"=w511) -> ("成功?"=w506:bool)  [unwired: 9 in]
                          n7940 = case shown="真" w506 {
                            tunnel: w509 -> [_ w518]
                            tunnel: w507 -> [_ w517]
                            frame False {
                              n7941 = local read "保持输入"() -> (w512:bool)
                              n7942 = case shown="假" w512 {
                                frame False {
                                n7943 = local read "同步_A1"() -> (w515:i32)
                                n7944 = local read "同步_A2"() -> (w513:i32)
                                n7945 = Increment(x=w515) -> (x+1=w516:i32)
                                n7946 = Increment(x=w513) -> (x+1=w514:i32)
                                n7947 = local write "同步_A2"(w514) -> ()
                                n7948 = local write "同步_A1"(w516) -> ()
                                }
                                frame True {
                                }
                              }
                            }
                            frame True {
                              n7949 = stacked-sequence {
                                tunnel: w518 -> [w523 _ _ _ _ _]
                                tunnel: w517 -> [_ w529 w548 _ _ _]
                                frame #0 {
                                n7950 = for {
                                tunnel: w523 -> [w526] mode=indexing
                                tunnel: [w525] -> w524 mode=indexing
                                n7951 = case shown="\"1\"" w526 {
                                tunnel: [FALSE TRUE] -> w525
                                frame "0", Default {
                                }
                                frame "1" {
                                }
                                }
                                }
                                n7952 = Boolean Array To Number ("布尔数组至数值转换")(Boolean array=w524) -> (number=w522:u16)
                                n7953 = Split Number(x=w522) -> (hi(x)=w519:u8, lo(x)=w520:u8)
                                n7954 = Build Array(w520, w519) -> (w521:u8[])
                                n7955 = call "DO"("dataIn(U8Array)"=w521) -> ()  [unwired: 2 in, 17 out]
                                }
                                frame #1 {
                                # "修改I/O标志"
                                n7956 = local read "同步_A1"() -> (w534:i32)
                                n7957 = Equal?(x=w534, y=4) -> (x = y?=w532:bool)
                                n7958 = Equal?(x=w534, y=5) -> (x = y?=w531:bool)
                                n7959 = Or(x=w532, y=w531) -> (x .or. y?=w530:bool)
                                n7960 = case shown="真" w530 {
                                tunnel: w529 -> [_ w536]
                                frame False {
                                }
                                frame True {
                                n7961 = stacked-sequence {
                                tunnel: w536 -> [w537 _ _ _]
                                frame #0 {
                                n7962 = Send Notification(notification="IOCheck" ("通知"), notifier=w537) -> ()  [unwired: 1 in, 2 out]
                                }
                                frame #1 {
                                n7963 = Wait Until Next ms Multiple(millisecond multiple=u32 10 ("毫秒倍数")) -> ()  [unwired: 1 out]
                                }
                                frame #2 {
                                n7964 = Build Array(u16 54, u16 0, u16 0) -> (w540:u16[])
                                n7965 = call "UDP发送.vi"("发送数据"=w540, "数据区字长"=u16 3, "报文类型"=u16 1285, "发送方标识"=u16 5397) -> ()  [unwired: 6 in, 1 out]
                                }
                                frame #3 {
                                n7966 = Wait (ms)(milliseconds to wait=u32 500 ("毫秒倍数")) -> ()  [unwired: 1 out]
                                }
                                }
                                }
                                }
                                }
                                frame #2 {
                                n7967 = Send Notification(notification="DICheck" ("通知"), notifier=w548) -> ()  [unwired: 1 in, 2 out]
                                }
                                frame #3 {
                                n7968 = Wait (ms)(milliseconds to wait=u32 5 ("等待时间（毫秒）")) -> ()  [unwired: 1 out]
                                }
                                frame #4 {
                                # "双向"
                                # "以太网请求反馈数据"
                                n7969 = Build Array(u16 1024, u16 1025, u16 54) -> (w557:u16[])
                                n7970 = call "UDP发送.vi"("发送数据"=w557, "数据区字长"=u16 3, "报文类型"=u16 2056, "发送方标识"=u16 5397) -> ()  [unwired: 6 in, 1 out]
                                }
                                frame #5 {
                                n7971 = local read "保持输入"() -> (w558:bool)
                                n7972 = case shown="假" w558 {
                                frame False {
                                n7973 = local read "同步_A1"() -> (w559:i32)
                                n7974 = Increment(x=w559) -> (x+1=w560:i32)
                                n7975 = local write "同步_A1"(w560) -> ()
                                }
                                frame True {
                                }
                                }
                                }
                              }
                            }
                          }
                        }
                      }
                    }
                  }
                }
              }
              n7976 = Wait Until Next ms Multiple(millisecond multiple=u32 5 ("毫秒倍数")) -> ()  [unwired: 1 out]
            }
          }
        }
        n7977 = local read "关闭？"() -> (w462:bool)
      }
      n7978 = Release Notifier(notifier=w205, error in (no error)=w204) -> ()  [unwired: 1 in, 3 out]
      n7979 = Obtain Notifier(name (unnamed)=w202, notification data type=w202) -> (notifier out=w199:refnum<notifier>, error out=w198:errorcluster)  [unwired: 2 in, 1 out]
      n7980 = while {
        tunnel: [w212] -> w201
        tunnel: [w211] -> w200
        tunnel: w199 -> [w210]
        tunnel: w198 -> [w209]
        stop <- w216 stop-if-true
        n7981 = Wait Until Next ms Multiple(millisecond multiple=u32 5 ("毫秒倍数")) -> ()  [unwired: 1 out]
        n7982 = Wait on Notification(notifier=w210, timeout in ms (-1)=20 ("超时毫秒(-1)"), error in (no error)=w209) -> (notifier out=w212:refnum<notifier>, notification=w208:string, error out=w211:errorcluster)  [unwired: 1 in, 1 out]
        n7983 = Equal?(x=w208, y="DICheck" ("通知")) -> (x = y?=w214:bool)
        n7984 = case shown="真" w214 {
          frame False {
          }
          frame True {
            n7985 = stacked-sequence {
              frame #0 {
                w222 = u16 6
                w230 = u16 5397
                # "错误报文类型"
                # "待定"
                n7986 = local read "保持输入"() -> (w223:bool)
                n7987 = Build Array(w230, u16 34952, u16 0 ("元素")) -> (w227:u16[])
                n7988 = case shown="假" w223 {
                  tunnel: [w233 w234] -> w224
                  frame False {
                    n7989 = local read "同步_A2"() -> (w233:i32)
                  }
                  frame True {
                    n7990 = local read "同步_A1"() -> (w234:i32)
                  }
                }
                n7991 = Build Array(w230, u16 2056, w222) -> (w231:u16[])
                n7992 = Add(x=w222, y=u16 4) -> (x+y=w220:u16)
                n7993 = call "UDP接收.vi"("匹配帧信息_异常"=w227, "长度"=w220, "匹配帧信息_正常"=w231) -> ("异常_找到?"=w226:bool, "接收超时?"=w225:bool, "接收的一帧数据"=w219:u16[], "正常_找到?"=w218:bool)  [unwired: 5 in]
                n7994 = case shown="真" w226 {
                  frame False {
                  }
                  frame True {
                    n7995 = call "对话框"("Message"="数字量输入返回数值异常") -> ()  [unwired: 9 in, 2 out]
                  }
                }
                n7996 = case shown="真" w225 {
                  frame False {
                  }
                  frame True {
                    n7997 = call "对话框2"("Message"="以太网接收数据超时失败") -> ()  [unwired: 9 in, 2 out]
                  }
                }
                n7998 = case shown="真" w218 {
                  tunnel: w219 -> [_ w238]
                  tunnel: w222 -> [_ w253]
                  tunnel: w224 -> [_ w237]
                  frame False {
                  }
                  frame True {
                    n7999 = To Long Integer(number=w253) -> (32bit integer=w242:i32)
                    n8000 = Array Subset(array=w238, index=3 ("索引"), length=w242) -> (w239:u16[])
                    n8001 = local read "数组_输入值"() -> (w244:enum16{"0", "1"}[][])
                    n8002 = local read "数组_选择?"() -> (w243:bool[][])
                    n8003 = call "更改输入顺序.vi"("输入数据"=w239) -> ("更改顺序后数据"=w241:u16[])  [unwired: 10 in]
                    n8004 = Index Array(array=w243, index (row)=w237) -> (element=w247:bool[])  [unwired: 1 in]
                    n8005 = Index Array(array=w244, index (row)=w237) -> (element=w246:enum16{"0", "1"}[])  [unwired: 1 in]
                    n8006 = Index Array(array=w241, index=w237) -> (element=w240:u16)
                    n8007 = Number To Boolean Array(number=w240) -> (Boolean array=w251:bool[])
                    n8008 = call "16路数字量输入判断.vi"("反馈值"=w251, "输入值"=w246, "是否选择"=w247) -> ("合格"=w248:bool, "结果"=w250:cluster{u32, u32}[][], "反馈值字符串"=w249:string[])  [unwired: 6 in]
                    n8009 = case shown="4" w237 {
                      tunnel: w250 -> [w255 w312 w349 w386 w423]
                      tunnel: w249 -> [w257 w293 w330 w366 w403]
                      frame 0, Default {
                        n8010 = local read "D_IN_1"() -> (w259:string[][])
                        n8011 = Replace Array Subset(array=w259, new element=w257, index (col)=2 ("禁用的索引 (列)")) -> (w256:string[][])  [unwired: 1 in]
